vi "DatabaseAPI-DisConnect.vi"(8 "error in":errorcluster, 11 "Database-API in":refnum<class "Database-API.lvclass">) -> (0 "error out":errorcluster, 3 "Database-API out":refnum<class "Database-API.lvclass">)   [LabVIEW 2014, in "Database-API.lvclass"]
uses:
  Database-API.lvclass
  Database-API.lvclass/Database-API.ctl
  <vilib>/addons/database/NI_Database_API.lvlib
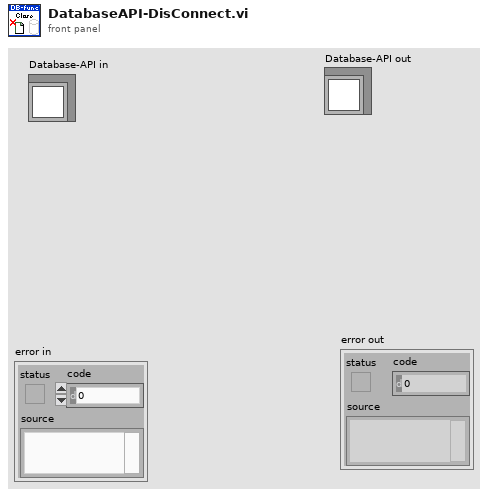
[diagram p1: front panel]
types:
  T1 = typedef "NI_Database_API.lvlib/Conn ObjectReference.ctl" = refnum<k1>
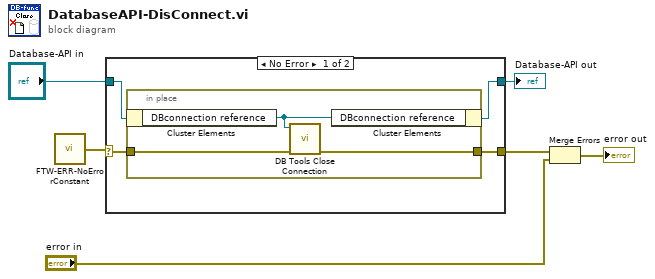
[diagram p0: block diagram]
diagram:
  n1 = call "FTW-ERR-NoErrorConstant.vi"() -> ("no error"=w5:errorcluster)
  n2 = case shown="No Error" w5 {
    selector: w5 -> [w10 w15]
    tunnel: [w9 w15] -> w3
    tunnel: [w7 w14] -> w4
    tunnel: "Database-API in" -> [w8 w14]
    frame No Error {
      n3 = in-place {
        in-place-border: w10 -> [w13]
        in-place-border: [w12] -> w9
        n4 = in-place-cluster #1(w8) -> ("DBconnection reference"=w11:T1)
        n5 = call <vilib>:"DB Tools Close Connection.vi"("error in (no error)"=w13, "connection reference"=w11) -> ("error out"=w12:errorcluster)  [unwired: 5 in]
        n6 = in-place-cluster #1("DBconnection reference"=w11) -> (w7:refnum<class "Database-API.lvclass">)
      }
    }
    frame Error {
    }
  }
  "Database-API out" <- w4
  n7 = Merge Errors(w3, "error in") -> (→"error out":errorcluster)
